vi "Instr_InitObject.vi"(8 "error in (no error)":errorcluster, 9 "Instrument Configuration":variant, 10 "GPIB Address":string, 11 "MultimeterControl in":refnum<class "MultimeterControl.lvclass">) -> (0 "error out":errorcluster, 3 "MultimeterControl out":refnum<class "MultimeterControl.lvclass">)   [LabVIEW 2019, in "MultimeterControl.lvclass"]
uses:
  MultimeterControl.lvclass
  InstrControl.lvclass
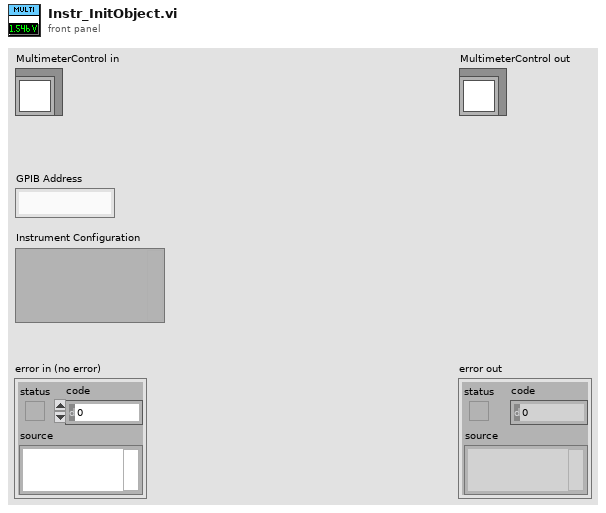
[diagram p1: front panel]
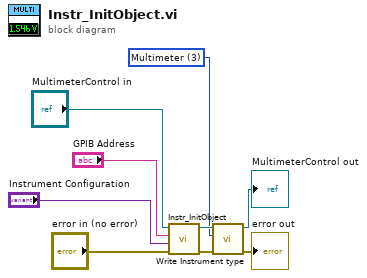
[diagram p0: block diagram]
diagram:
  w2 = u16 3 items=["Supply", "LCR", "Switching", "Multimeter"] ("Instrument type")
  n1 = call-parent "Instr_InitObject.vi"("error in (no error)"="error in (no error)", "Instrument Configuration"="Instrument Configuration", "GPIB Address"="GPIB Address", "InstrControl in"="MultimeterControl in") -> ("error out"=w6:errorcluster, "InstrControl out"=w4:refnum<class "MultimeterControl.lvclass">)  [unwired: 6 in]
  n2 = call-dynamic "Write Instrument type.vi"("error in (no error)"=w6, "Instrument type"=w2, "InstControl in"=w4) -> ("error out"=→"error out":errorcluster, "InstControl out"=→"MultimeterControl out":refnum<class "MultimeterControl.lvclass">)  [unwired: 7 in]
